vi "Initialize.vi"   [LabVIEW 2023, in "RTL-SDR.lvlib"]
uses:
  RTL-SDR.lvlib
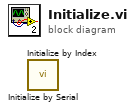
[diagram p0: block diagram]
diagram:
  n1 = call "Initialize by Serial.vi"() -> ()  [unwired: 10 in, 2 out]
  n2 = call "Initialize by Index.vi"() -> ()  [unwired: 10 in, 2 out]
